vi "App Loop.vi"() -> ()   [LabVIEW 2018]
uses:
  Controls/App Global Mode.ctl
  <vilib>/NI_Real-Time Target Support.lvlib
panel:
  in  "Login":bool
types:
  T1 = typedef "App Global Mode.ctl" = enum16{"Read", "Write Client", "Write Login"}
  T2 = typedef "LVRemotePanelConnectionsTypeDef.ctl" = cluster{"VI Name":string, "Remote":string, "UserName":string, "Port":i32, "Status":enum32{"Viewing", "Waiting For Control", "Controlling"}, "Create Time":timestamp, "Status Time":timestamp, "Control End Time":timestamp}[]
  T3 = typedef "NI_Real-Time Target Support.lvlib/RT CPU Load.ctl" = cluster{"Total (%)":dbl, "Time Critical (%)":dbl, "Timed Structures (%)":dbl, "High (%)":dbl, "Above Normal (%)":dbl, "Normal (%)":dbl, "Background (%)":dbl, "Idle (%)":dbl, "ISR (%)":dbl}
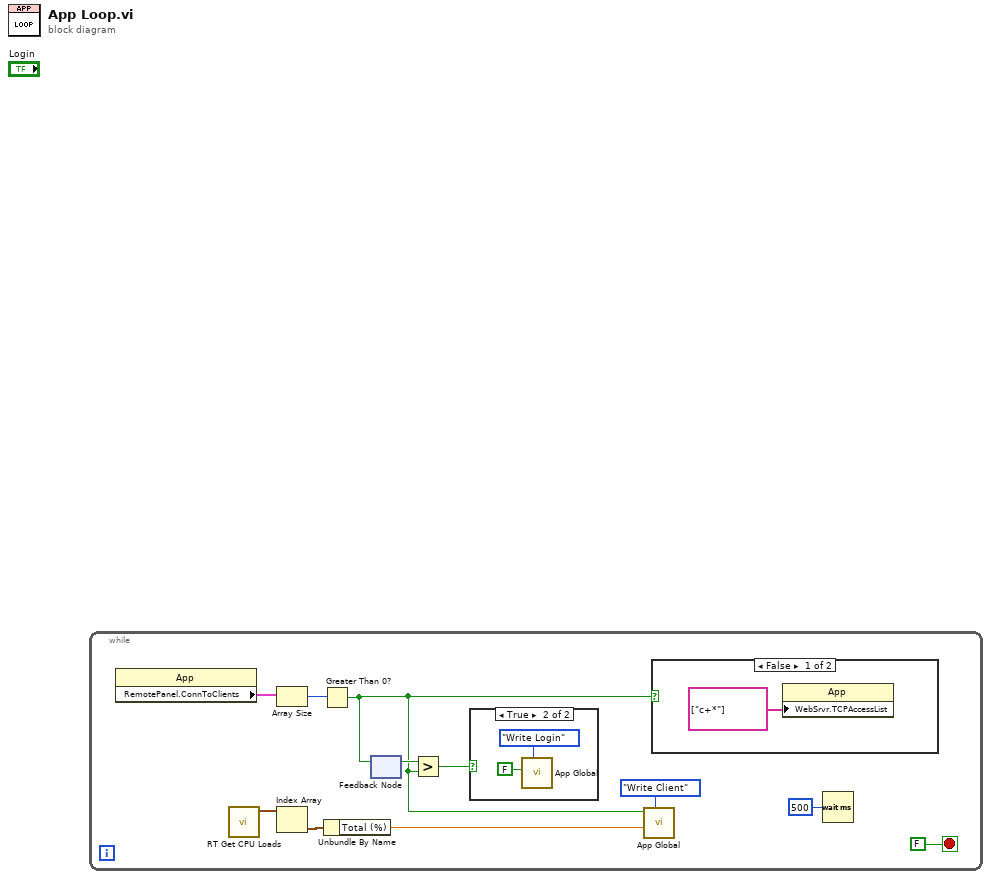
[diagram p0: block diagram]
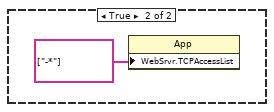
[diagram p2: hidden frame]
diagram:
  n1 = while {
    stop <- FALSE stop-if-true
    n2 = property class="App"() -> ("RemotePanel.ConnToClients"=w6:T2)  [unwired: 2 in, 2 out]
    n3 = call <vilib>:"RT Get CPU Loads.vi"() -> ("CPU loads"=w4:T3[])  [unwired: 10 in, 1 out]
    n4 = Array Size(array=w6) -> (size(s)=w9:i32)
    n5 = Index Array(array=w4) -> (element=w5:T3)  [unwired: 1 in]
    n6 = Greater Than 0?(x=w9) -> (x > 0?=w2:bool)
    n7 = Unbundle By Name(w5) -> ("Total (%)"=w3:dbl)
    n8 = feedback #1() -> (w8:bool)  [unwired: 1 in]
    n9 = feedback-in #1(w2) -> ()
    n10 = Greater?(x=w8, y=w2) -> (0:w7:bool)
    n11 = case shown="True" w7 {
      frame False {
      }
      frame True {
        n12 = call "App Global.vi"("Mode"=App_Global_Mode."Write Login", "Login"=FALSE) -> ()  [unwired: 7 in, 3 out]
      }
    }
    n13 = call "App Global.vi"("Mode"=App_Global_Mode."Write Client", "CPU Usage:"=w3, "Client?"=w2) -> ()  [unwired: 6 in, 3 out]
    n14 = case shown="False" w2 {
      frame False {
        n15 = property class="App"("WebSrvr.TCPAccessList"=string[] ["c+*"] ("Web Server:TCP/IP Access List")) -> ()  [unwired: 2 in, 2 out]
      }
      frame True {
        n16 = property class="App"("WebSrvr.TCPAccessList"=string[] ["-*"] ("Web Server:TCP/IP Access List")) -> ()  [unwired: 2 in, 2 out]
      }
    }
    n17 = Wait (ms)(milliseconds to wait=u32 500) -> ()  [unwired: 1 out]
  }
